vi "Forget Subscriber.vi"(8 "error in (no error)":errorcluster, 10 "Subscription Policy":T1, 11 "IBusMonitor In":refnum<class "IBusMonitor.lvclass">) -> (0 "error out":errorcluster, 3 "IBusMonitor Out":refnum<class "IBusMonitor.lvclass">)   [LabVIEW 2020, in "MVA Framework.lvlib" / "MonitoredMediator.lvlib" / "IBusMonitor.lvclass"]
uses:
  IBusMonitor.lvclass
  IMediator/ISubscriptionPolicy/ISubscriptionPolicy Reference.ctl
  IMediator/ISubscriptionPolicy/ISubscriptionPolicy.lvclass
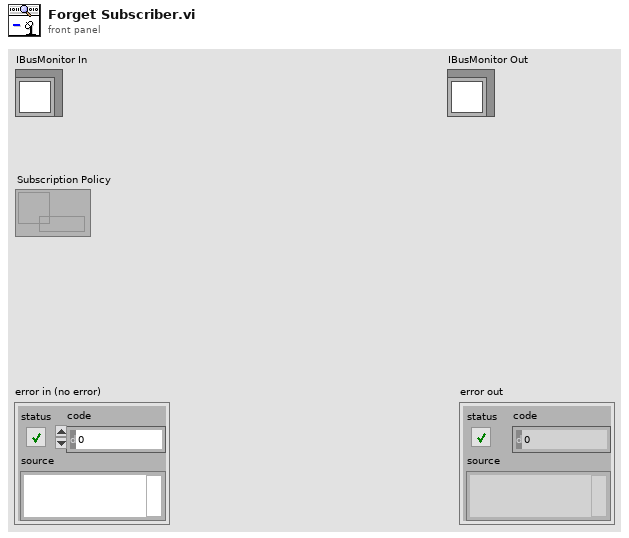
[diagram p1: front panel]
types:
  T1 = typedef "MVA Framework.lvlib/IMediator.lvlib/ISubscriptionPolicy.lvclass/ISubscriptionPolicy Reference.ctl" = refnum<data-value>
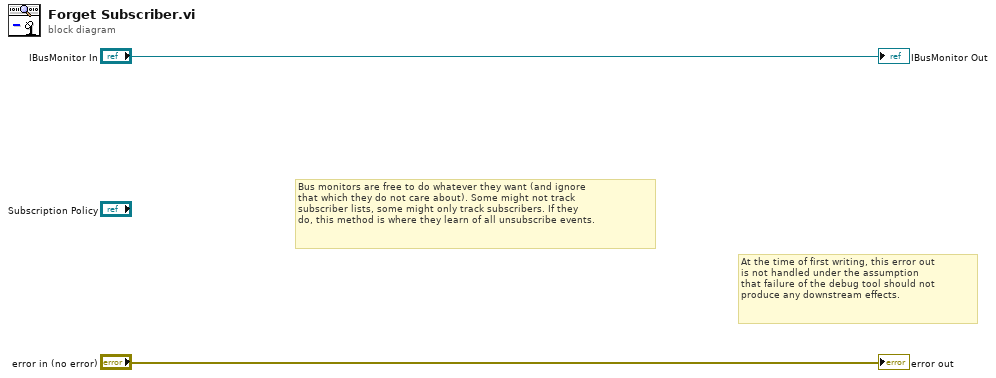
[diagram p0: block diagram]
diagram:
  # "At the time of first writing, this error out\nis not handled under the assumption\nthat failure of the debug tool should not\nproduce any downstream effects."
  # "Bus monitors are free to do whatever they want (and ignore\nthat which they do not care about). Some might not track\nsubscriber lists, some might only track subscribers. If they\ndo, this method is where they learn of all unsubscribe events."
  "error out" <- "error in (no error)"
  "IBusMonitor Out" <- "IBusMonitor In"
